vi "qn_initialStepsize.vi"(4 "Gamma":dbl=2.0, 6 "F(X)":dbl=nan, 7 "function and data":T1, 8 "error in (no error)":errorcluster, 9 "Direction":dbl[](array[numeric]), 10 "X":dbl[](array[numeric])) -> (0 "error out":errorcluster, 1 "number of function calls":i32, 3 "s":dbl)   [LabVIEW 2020, in "NI_Gmath.lvlib"]
uses:
  NI_Gmath.lvlib
  ucno_user function ref and data.ctl
  ucno_user objective function ref.ctl
panel:
  out "iter count":i32
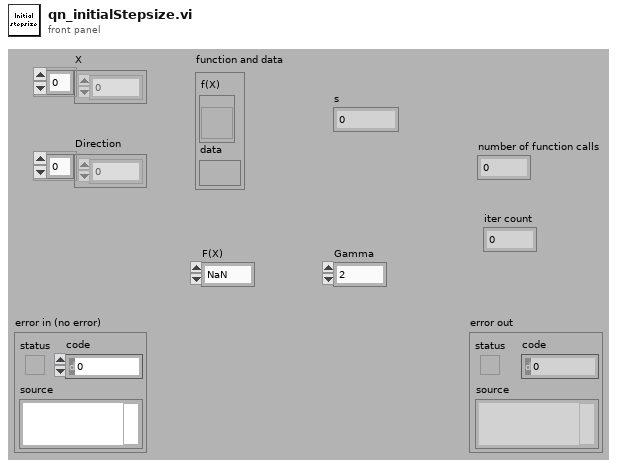
[diagram p1: front panel]
types:
  T1 = typedef "NI_Gmath.lvlib/ucno_user function ref and data.ctl" = cluster{"f(X)":T2, "data":variant}
  T2 = typedef "NI_Gmath.lvlib/ucno_user objective function ref.ctl" = refnum<vi>
  T3 = cluster{"objective function":bool, "gradient":bool}
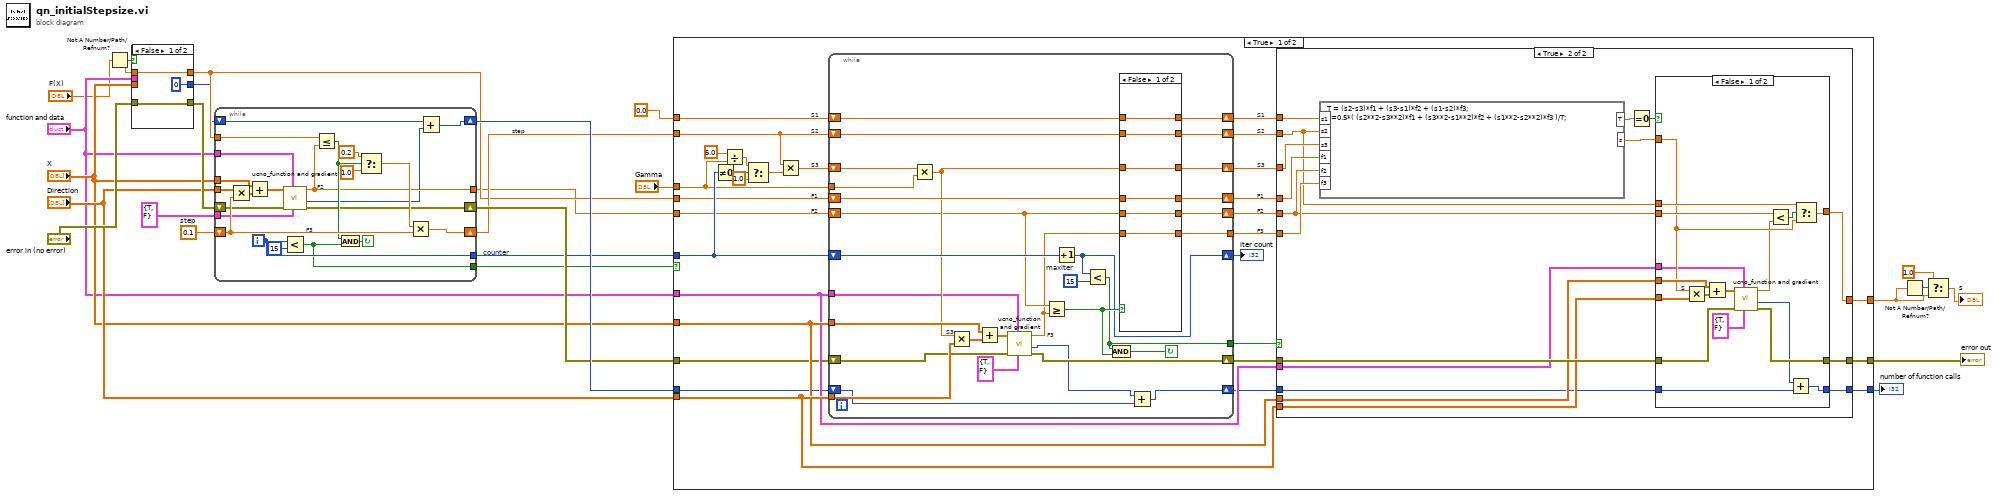
[diagram p0: block diagram]
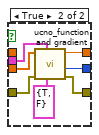
[diagram p2: hidden frame]
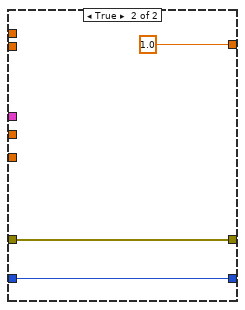
[diagram p4: hidden frame]
diagram:
  w20 = 0.1  # step
  # "step"
  # "counter"
  n1 = Not A Number/Path/Refnum?(number/path/refnum="F(X)") -> (NaN/Path/Refnum?=w14:bool)
  n2 = case shown="False" w14 {
    tunnel: "X" -> [_ w35]
    tunnel: "function and data" -> [_ w30]
    tunnel: "F(X)" -> [w28 _]
    tunnel: [w28 w34] -> w10
    tunnel: "error in (no error)" -> [w27 w32]
    tunnel: [w27 w33] -> w23
    tunnel: [0 ("number of function calls") w29] -> w2
    frame False {
    }
    frame True {
      n3 = call "ucno_function and gradient.vi"("output control"=T3 {"objective function"=TRUE, "gradient"=FALSE}, "function and data"=w30, "error in (no error)"=w32, "X"=w35) -> ("error out"=w33:errorcluster, "number of function calls"=w29:i32, "f(X)"=w34:dbl)  [unwired: 4 in, 1 out]
    }
  }
  n4 = while {
    tunnel: w10 -> [w58]
    shift-right: [w57] -> w16
    shift-left: w20 -> [w49]
    tunnel: "Direction" -> [w54]
    tunnel: "X" -> [w52]
    tunnel: "function and data" -> [w42]
    tunnel: [w51] -> w21
    tunnel: [w50] -> w19
    tunnel: [w41] -> w9
    shift-right: [w43] -> w22
    shift-left: w23 -> [w44]
    tunnel: T3 {"objective function"=TRUE, "gradient"=FALSE} ("output control") -> [w39]
    shift-right: [w36] -> w25
    shift-left: w2 -> [w37]
    i -> [w51]
    stop <- w55 continue-if-true
    # "F2"
    # "F3"
    n5 = Multiply(x=w54, y=w49) -> (x*y=w53:dbl[])
    n6 = Add(x=w52, y=w53) -> (x+y=w40:dbl[])
    n7 = call "ucno_function and gradient.vi"("output control"=w39, "function and data"=w42, "error in (no error)"=w44, "X"=w40) -> ("error out"=w43:errorcluster, "number of function calls"=w38:i32, "f(X)"=w41:dbl)  [unwired: 4 in, 1 out]
    n8 = Less?(x=w51, y=15) -> (x < y?=w50:bool)
    n9 = Less Or Equal?(x=w58, y=w41) -> (x <= y?=w48:bool)
    n10 = And(x=w48, y=w50) -> (x .and. y?=w55:bool)
    n11 = Select(t=0.2 ("y"), s=w48, f=1.0 ("y")) -> (s? t:f=w45:dbl)
    n12 = Multiply(x=w45, y=w49) -> (x*y=w57:dbl)
    n13 = Add(x=w37, y=w38) -> (x+y=w36:i32)
  }
  n14 = case shown="True" w19 {
    tunnel: [w74 w172] -> w5
    tunnel: "X" -> [w67 _]
    tunnel: "Direction" -> [w68 _]
    tunnel: w9 -> [w87 _]
    tunnel: w21 -> [w88 _]
    tunnel: "Gamma" -> [w77 _]
    tunnel: 0.0 -> [w86 _]
    tunnel: w16 -> [w79 w172]
    tunnel: w10 -> [w85 _]
    tunnel: "function and data" -> [w66 _]
    tunnel: w22 -> [w64 w171]
    tunnel: [w62 w171] -> w4
    tunnel: w25 -> [w60 w170]
    tunnel: [w59 w170] -> w1
    frame True {
      # "F3"
      # "F2"
      # "F1"
      # "S3"
      # "S2"
      # "S1"
      # "F2"
      # "F1"
      # "S3"
      # "S2"
      # "S1"
      n15 = Not Equal To 0?(x=w88) -> (x != 0?=w80:bool)
      n16 = Divide(x=5.0, y=w77) -> (x/y=w83:dbl)
      n17 = Select(t=w83, s=w80, f=1.0) -> (s? t:f=w81:dbl)
      n18 = Multiply(x=w79, y=w81) -> (x*y=w78:dbl)
      n19 = while {
        tunnel: w67 -> [w159]
        tunnel: w68 -> [w158]
        shift-right: [w138] -> w65
        shift-left: w88 -> [w156]
        shift-right: [w155] -> w75
        shift-left: w78 -> [w151]
        tunnel: w77 -> [w152]
        shift-right: [w142] -> w73
        shift-left: w86 -> [w146]
        shift-right: [w143] -> w72
        shift-left: w79 -> [w147]
        shift-right: [w140] -> w70
        shift-left: w87 -> [w145]
        shift-right: [w141] -> w71
        shift-left: w85 -> [w149]
        tunnel: [w144] -> w76
        tunnel: [w139] -> w69
        tunnel: w66 -> [w136]
        shift-right: [w133] -> w63
        shift-left: w64 -> [w134]
        shift-right: [w130] -> w61
        shift-left: w60 -> [w129]
        stop <- w153 continue-if-true
        w154 = 15  # maxiter
        # "S3"
        # "F3"
        n20 = Multiply(x=w151, y=w152) -> (x*y=w148:dbl)
        n21 = Multiply(x=w148, y=w158) -> (x*y=w157:dbl[])
        n22 = Add(x=w159, y=w157) -> (x+y=w135:dbl[])
        n23 = call "ucno_function and gradient.vi"("output control"=T3 {"objective function"=TRUE, "gradient"=FALSE}, "function and data"=w136, "error in (no error)"=w134, "X"=w135) -> ("error out"=w133:errorcluster, "number of function calls"=w131:i32, "f(X)"=w137:dbl)  [unwired: 4 in, 1 out]
        n24 = Greater Or Equal?(x=w145, y=w137) -> (x >= y?=w150:bool)
        n25 = Increment(x=w156) -> (x+1=w138:i32)
        n26 = Less?(x=w138, y=w154) -> (x < y?=w144:bool)
        n27 = And(x=w144, y=w150) -> (x .and. y?=w153:bool)
        n28 = case shown="False" w150 {
          tunnel: [w165 w168] -> w155
          tunnel: w149 -> [w162 _]
          tunnel: w137 -> [w160 w166]
          tunnel: w148 -> [w165 w168]
          tunnel: w147 -> [w164 w169]
          tunnel: w146 -> [w163 _]
          tunnel: w145 -> [w161 w167]
          tunnel: [w164 w168] -> w143
          tunnel: [w163 w169] -> w142
          tunnel: [w162 w167] -> w141
          tunnel: [w161 w166] -> w140
          tunnel: [w160 w166] -> w139
          frame False {
          }
          frame True {
          }
        }
        n29 = Add(x=w131, y=w129) -> (x+y=w130:i32)
      }
      "iter count" <- w65
      n30 = case shown="True" w76 {
        tunnel: w75 -> [w91 w106]
        tunnel: [w91 w101] -> w74
        tunnel: w73 -> [_ w107]
        tunnel: w72 -> [_ w96]
        tunnel: w71 -> [_ w105]
        tunnel: w70 -> [_ w97]
        tunnel: w69 -> [_ w104]
        tunnel: w68 -> [_ w98]
        tunnel: w67 -> [_ w99]
        tunnel: w66 -> [_ w95]
        tunnel: w63 -> [w90 w108]
        tunnel: [w90 w94] -> w62
        tunnel: w61 -> [w89 w93]
        tunnel: [w89 w92] -> w59
        frame False {
        }
        frame True {
          n31 = formula code="T = (s2-s3)*f1 + (s3-s1)*f2 + (s1-s2)*f3;\ns=0.5*( (s2**2-s3**2)*f1 + (s3**2-s1**2)*f2 + (s1**2-s2**2)*f3 )/T;"("s1"=w107, "s2"=w96, "s3"=w106, "f1"=w105, "f2"=w97, "f3"=w104) -> ("s"=w100:dbl, "T"=w103:dbl)
          n32 = Equal To 0?(x=w103) -> (x = 0?=w102:bool)
          n33 = case shown="False" w102 {
            tunnel: [w118 1.0] -> w101
            tunnel: w100 -> [w119 _]
            tunnel: w99 -> [w124 _]
            tunnel: w98 -> [w123 _]
            tunnel: w97 -> [w122 _]
            tunnel: w96 -> [w120 _]
            tunnel: w95 -> [w115 _]
            tunnel: w108 -> [w117 w127]
            tunnel: [w116 w127] -> w94
            tunnel: w93 -> [w110 w126]
            tunnel: [w109 w126] -> w92
            frame False {
              # "S"
              n34 = Multiply(x=w119, y=w123) -> (x*y=w125:dbl[])
              n35 = Add(x=w124, y=w125) -> (x+y=w113:dbl[])
              n36 = call "ucno_function and gradient.vi"("output control"=T3 {"objective function"=TRUE, "gradient"=FALSE}, "function and data"=w115, "error in (no error)"=w117, "X"=w113) -> ("error out"=w116:errorcluster, "number of function calls"=w111:i32, "f(X)"=w114:dbl)  [unwired: 4 in, 1 out]
              n37 = Less?(x=w122, y=w114) -> (x < y?=w121:bool)
              n38 = Add(x=w111, y=w110) -> (x+y=w109:i32)
              n39 = Select(t=w120, s=w121, f=w119) -> (s? t:f=w118:dbl)
            }
            frame True {
            }
          }
        }
      }
    }
    frame False {
    }
  }
  "error out" <- w4
  "number of function calls" <- w1
  n40 = Not A Number/Path/Refnum?(number/path/refnum=w5) -> (NaN/Path/Refnum?=w8:bool)
  n41 = Select(t=1.0, s=w8, f=w5) -> (s? t:f=→"s":dbl)
